vi "Engine Simulation Global.vi"() -> ()   [LabVIEW 2011, in "Engine Simulation Shared.lvlib"]
uses:
  Engine Simulation Shared.lvlib
panel:
  in  "TAB-Strings":enum32{"GUIDS", "Properties", "Sysdef Tree"}(tab)=enum."Properties"
  in  "Crank and Cams GUID":string="B8A54196-A3EC-62F7-D181-DF8C7E0BE69D"
  in  "N Teeth M Missing GUID":string="D13AE4FE-5D80-B0CC-FDA0-9157C9A149E5"
  in  "Fully Custom Collection GUID":string="F50F9943-5E77-7915-BB8D-E6902279B28E"
  in  "Fully Custom GUID":string="C620946F-22B4-9CF6-4F15-9C7CC7CA9D8C"
  in  "ECU Events GUID":string="C0F2F8B4-F3D7-60C5-FF9F-3CDFC1FB32F6"
  in  "ECU Event GUID":string="0C39D0EB-6C13-AC47-ACCA-A16625DA2D25"
  in  "Data Replay Loop GUID":string="A6C5F3D6-D595-FB51-CC0F-A3E187312E4C"
  in  "Data Replay GUID":string="A1C69264-1A23-45C8-CFFF-4B9A0433C19C"
  in  "APU GUID":string="164D4EF3-DDDB-483A-8ED9-6596F8ED3FBF"
  in  "Channel Del Prot GUID":string="7C871B01-1266-4EDB-A195-BFBED06C858B"
  in  "Main Page GUID":string="981B5D80-125D-3755-C95E-D7EA1B6DEE7D"
  in  "Status Channels Page GUID":string="4B53A2D5-350B-49B1-8BEC-61C7CFC9989F"
  in  "TAB-Properties":T1(tab)=enum."Data Replay"
  in  "FPGA Type":string="FPGA Type"
  in  "FPGA Path":string="FPGA Path"
  in  "FPGA Name":string="FPGA Name"
  in  "FPGA Reference":string="FPGA Reference"
  in  "VSFPGA Win Path":string="VSFPGA Win Path"
  in  "FPGA RT Path":string="FPGA RT Path"
  in  "Engine Sim Config":string="Engine Sim Config"
  in  "APU.SlewRate":string="APU.SlewRate"
  in  "APU Component":string="APU Component"
  in  "NTeeth.CycleAngle?":string="NTeeth.CycleAngle?"
  in  "NTeeth Settings":string="NTeeth Settings"
  in  "FullyCustom Comm Mode":string="FullyCustom Comm Mode"
  in  "FullyCustom Profiles":string="FullyCustom Profiles"
  in  "FullyCustom Settings":string="FullyCustom Settings"
  in  "FullyCustom.CycleAngle?":string="FullyCustom.CycleAngle?"
  in  "FullyCustomColl Settings":string="FullyCustomColl Settings"
  in  "Profiles Offset":string="Profiles Offset"
  in  "EventParentRate?":string="EventParentRate?"
  in  "EventLoopRate":string="EventLoopRate"
  in  "ECUEvent Components":string="ECUEvent Components"
  in  "ECUEvent Measurements":string="ECUEvent Measurements"
  in  "DataReplayLoop.#OfReplays":string="DataReplayLoop.#OfReplays"
  in  "DataReplayLoop.ReplayMem#s":string="DataReplayLoop.ReplayMem#s"
  in  "DataReplayLoop.ReplayOptionals":string="DataReplayLoop.ReplayOptionals"
  in  "DataReplayLoop.ReplayNames":string="DataReplayLoop.ReplayNames"
  in  "DataReplay.AngleOffset":string="DataReplay.AngleOffset"
  in  "DataReplay.VOverride":string="DataReplay.VOverride"
  in  "DataReplay.ReverseNegate":string="DataReplay.ReverseNegate"
  in  "DataReplay.Reverse":string="DataReplay.Reverse"
  in  "DataReplay.FileLength":string="DataReplay.FileLength"
  in  "DataReplay.FileOffset":string="DataReplay.FileOffset"
  in  "DataReplay.FileMethod":string="DataReplay.FileMethod"
  in  "DataReplay.FileDataPlugin":string="DataReplay.FileDataPlugin"
  in  "DataReplay.FileChannel":string="DataReplay.FileChannel"
  in  "DataReplay.FileGroup":string="DataReplay.FileGroup"
  in  "DataReplay.File":string="DataReplay.File"
  in  "DataReplay.MissingLocation":string="DataReplay.MissingLocation"
  in  "DataReplay.VatCutoff":string="DataReplay.VatCutoff"
  in  "DataReplay.VatMax":string="DataReplay.VatMax"
  in  "DataReplay.AngleRef":string="DataReplay.AngleRef"
  in  "DataReplay.MaxSpeed":string="DataReplay.MaxSpeed"
  in  "DataReplay.CutoffSpeed":string="DataReplay.CutoffSpeed"
  in  "DataReplay.DACBits":string="DataReplay.DACBits"
  in  "DataReplay.MemSize":string="DataReplay.MemSize"
  in  "DataReplayLoop.Rate":string="DataReplayLoop.Rate"
  in  "DataReplay.Mem#":string="DataReplay.Mem#"
  in  "CrankCams.DataReplayLoopNames":string="CrankCams.DataReplayLoopNames"
  in  "CrankCams.#DataReplayLoops":string="Data Replay Loop Components"
  in  "FullyCustom Components":string="FullyCustom Components"
  in  "NTeeth Components":string="NTeeth Components"
  in  "TAB-Channel Names":enum32{"Data Replay"}(tab)
  in  "Data Replay Chans":string[](array[string])=["Offset"]
  in  "Event Chans":string[](array[string])=["Time Duration", "Start Angle", "End Angle", "Angle Duration"]
  in  "Status Section Name":string="Status Channels"
  in  "Status Chans Descrip":string[](array[string])=["The number of times the Engine Simulation Loop reported being late", "The duration of the Engine Simulation Loop in nanoseconds", "Error Code generated by the engine simulation cusom device. A non zero value could indicate failure."]
  in  "Status Chans":string[](array[string])=["ES Count", "ES Loop Duration", "Error Code"]
  in  "DataReplay.VoltageChans":string[](array[string])=["Enable voltage override", "Voltage slope", "Voltage intercept"]
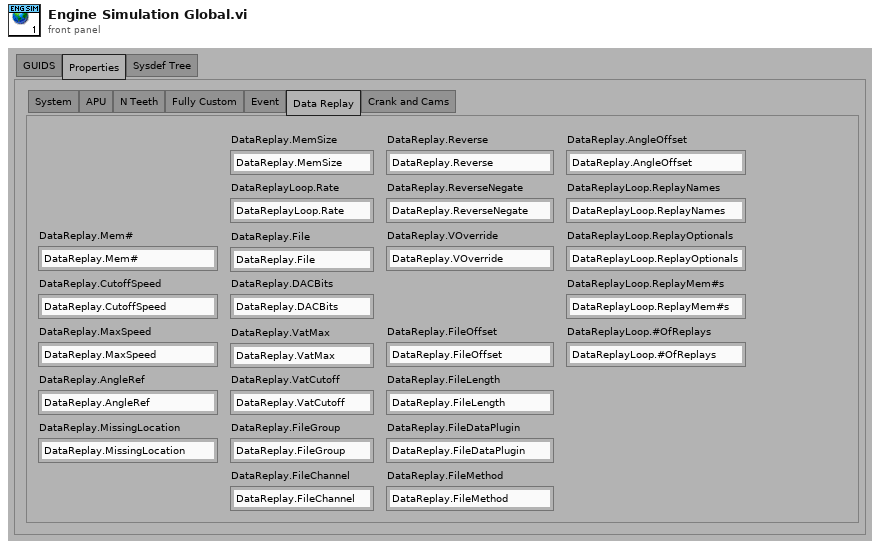
[diagram p1: front panel]
types:
  T1 = enum32{"System", "APU", "N Teeth", "Fully Custom", "Event", "Data Replay", "Crank and Cams"}
diagram:
